vi "_Read File Header.vi"(5 "error in (no error)":errorcluster, 7 "File Size":i64, 8 "File Refnum In":refnum<file>) -> (0 "error out":errorcluster, 1 "Version":i32, 2 "Offsets":i64[](array[numeric]), 3 "File Refnum Out":refnum<file>, 4 "AcqMethod":T1[](array[typedef]) {"ScanType" format="%#.6g"; "Mass Range"."Res" items=["High/High", "Medium/Medium", "Low/Low", "High/Medium", "High/Low", "Medium/High", "Medium/Low", "Low/High", "Low/Medium"]})   [LabVIEW 2015]
uses:
  Type/_XML Expt.ctl
  Type/_XML Lens.ctl
  Type/_Mass Range Property.ctl
  Type/_Mass Range Parameters.ctl
  Type/_RT Res Type.ctl
  Type/_GUI Method.ctl
  Type/_Lens Property.ctl
  Type/_Run Mode.ctl
  Configuration/_Global Configuration.vi
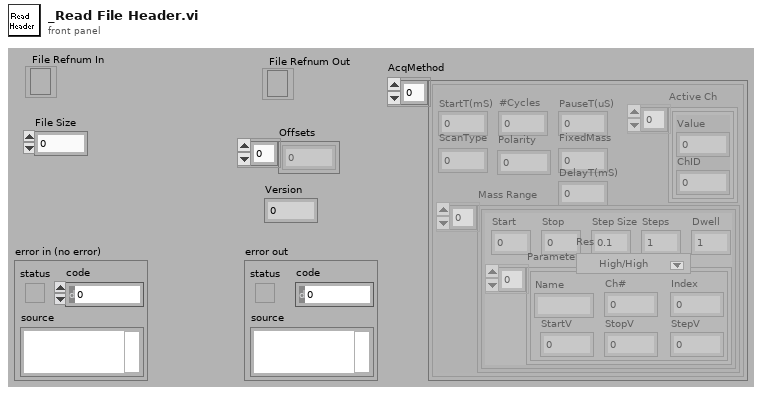
[diagram p1: front panel]
types:
  T1 = typedef "_XML Expt.ctl" = cluster{"StartT(mS)":i32, "#Cycles":i32, "PauseT(uS)":i32, "ScanType":i32, "Polarity":u8, "FixedMass":dbl, "DelayT(mS)":i32, "Active Ch":T2[], "Mass Range":T3[]}
  T2 = typedef "_XML Lens.ctl" = cluster{"Value":dbl, "ChID":u8}
  T3 = typedef "_Mass Range Property.ctl" = cluster{"Start":dbl, "Stop":dbl, "Step Size":dbl, "Steps":i32, "Dwell":dbl, "Parameters":T4[], "Res":T5}
  T4 = typedef "_Mass Range Parameters.ctl" = cluster{"Name":string, "Ch#":u8, "StartV":dbl, "StopV":dbl, "StepV":dbl, "Index":u8}
  T5 = typedef "_RT Res Type.ctl" = u16
  T6 = typedef "_GUI Method.ctl" = cluster{"Lenses":T7[], "Mass Ranges":T3[], "Acquire":bool, "MCA":bool, "Q1DC EN":bool, "Q1 POL":bool, "Q3 POL":bool, "Q1 RF  EN":bool, "Averaging":bool, "Log Scale":bool, "CPS":bool, "Unit":bool, "Data Path":path, "Run Mode":T8, "Fixed Mass (amu)":dbl, "Q3DC EN":bool, "Q3 RF  EN":bool, "Negative":bool}
  T7 = typedef "_Lens Property.ctl" = cluster{"Scan Type":u8, "Scans":i32, "Time 1":dbl, "Time 2":dbl, "Value 1":dbl, "Value 2":dbl, "Step Size":dbl}
  T8 = typedef "_Run Mode.ctl" = enum16{"MRM (Q1/Q2)", "Q1 Scan", "Q1 SRM", "Q2 Scan", "Q2 SRM", "Product Scan", "Precursor Scan", "Neutral Loss", "Neutral Gain"}
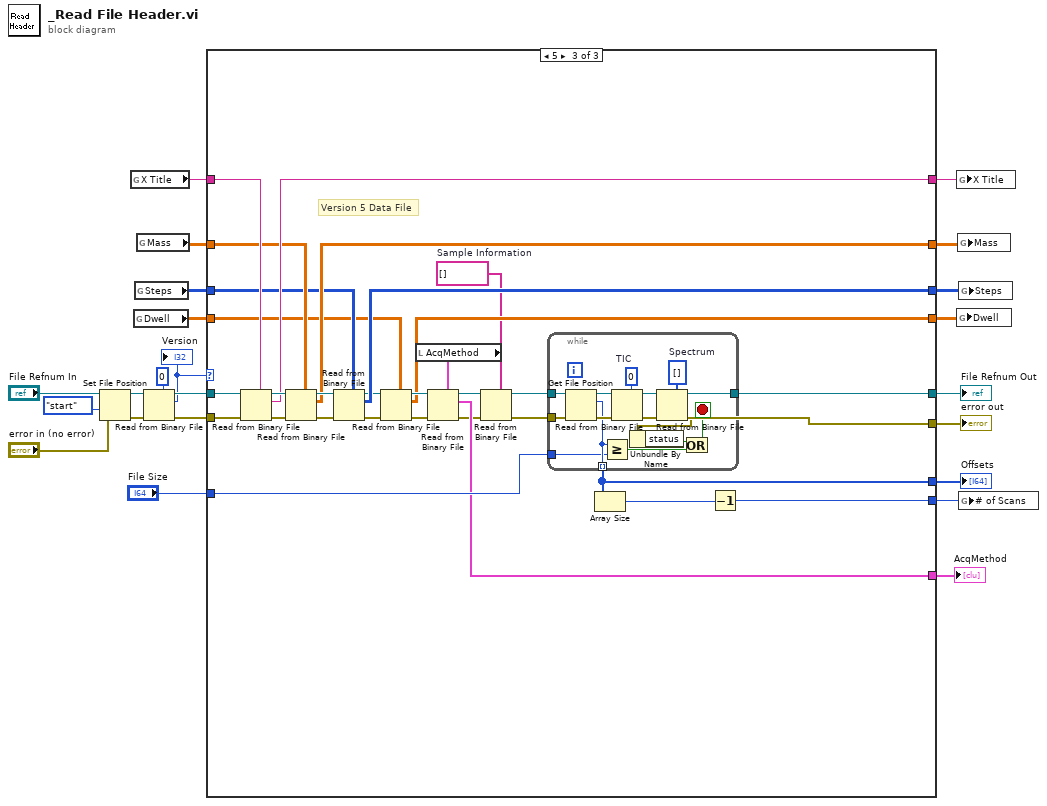
[diagram p0: block diagram]
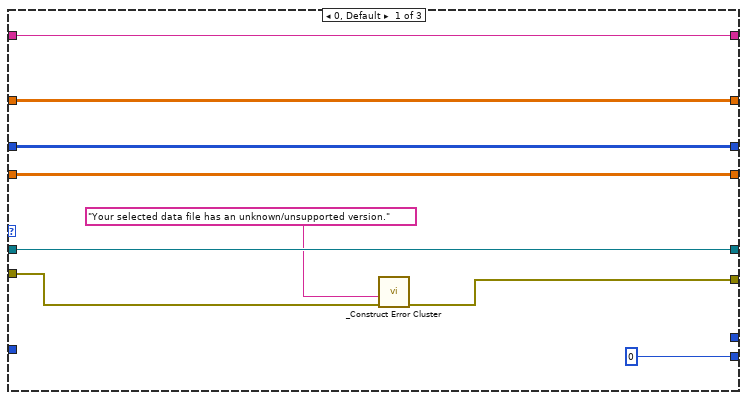
[diagram p2: hidden frame]
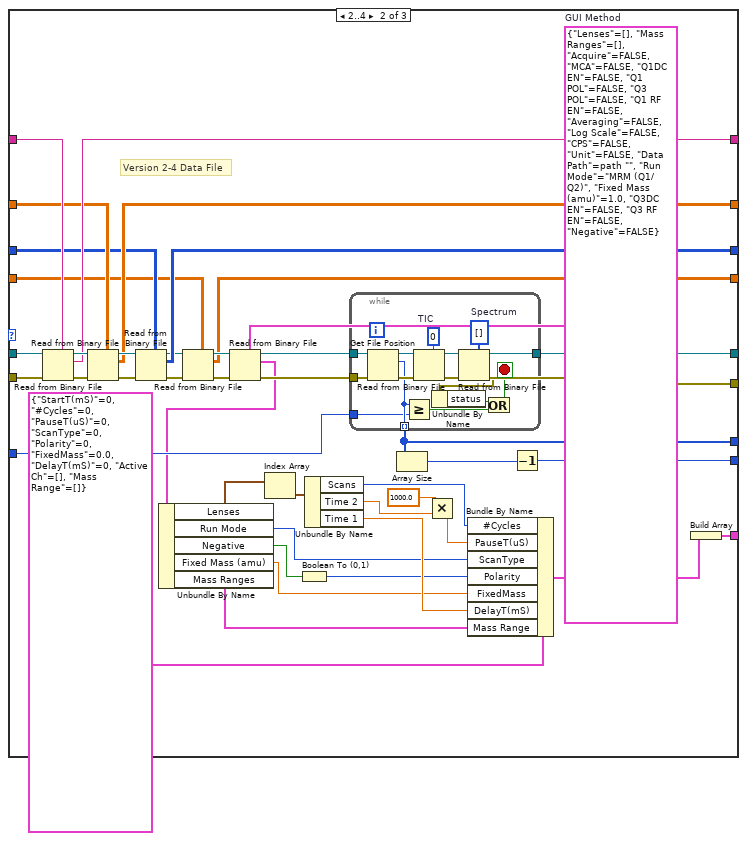
[diagram p3: hidden frame]
diagram:
  n1 = Set File Position(refnum="File Refnum In", from (0:start)=enum16{"start", "end", "current"}."start" ("pos mode (0:2)"), error in="error in (no error)") -> (refnum out=w16:refnum<file>, error out=w15:errorcluster)  [unwired: 1 in]
  n2 = global read "_Global Configuration.vi" "X Title"() -> (w7:string)
  n3 = global read "_Global Configuration.vi" "Dwell"() -> (w4:dbl[][])
  n4 = global read "_Global Configuration.vi" "Steps"() -> (w5:i32[][])
  n5 = global read "_Global Configuration.vi" "Mass"() -> (w6:dbl[][])
  n6 = Read from Binary File(5:0 ("pos offset (0)"), 8:w15, 11:w16) -> (0:w21:errorcluster, 2:w14:i32, 3:w20:refnum<file>)  [unwired: 4 out]
  "Version" <- w14
  n7 = case shown="5" w14 {
    tunnel: w21 -> [w28 w72 w117]
    tunnel: w20 -> [w29 w71 w116]
    tunnel: [w31 w68 w113] -> w17
    tunnel: [w32 w66 w111] -> w13
    tunnel: [0 w51 w98] -> w12
    tunnel: [w29 w55 w101] -> w11
    tunnel: [w26 w54 w92] -> w10
    tunnel: "File Size" -> [_ w50 w97]
    tunnel: [w30 w67 w112] -> w8
    tunnel: w7 -> [w32 w65 w110]
    tunnel: w6 -> [w31 w64 w109]
    tunnel: w5 -> [w30 w63 w108]
    tunnel: w4 -> [w25 w57 w103]
    tunnel: [w25 w56 w102] -> w3
    tunnel: [_ w53 w100] -> w2
    tunnel: [_ w46 w96] -> w1
    frame 0, Default {
      n8 = call "_Construct Error Cluster.vi"("error in"=w28, "reason"="Your selected data file has an unknown/unsupported version.") -> ("error out"=w26:errorcluster)  [unwired: 2 in, 3 out]
    }
    frame 2..4 {
      w49 = T6 {"Lenses"=[], "Mass Ranges"=[], "Acquire"=FALSE, "MCA"=FALSE, "Q1DC EN"=FALSE, "Q1 POL"=FALSE, "Q3 POL"=FALSE, "Q1 RF  EN"=FALSE, "Averaging"=FALSE, "Log Scale"=FALSE, "CPS"=FALSE, "Unit"=FALSE, "Data Path"=path "", "Run Mode"=enum."MRM (Q1/Q2)", "Fixed Mass (amu)"=1.0, "Q3DC EN"=FALSE, "Q3 RF  EN"=FALSE, "Negative"=FALSE}  # GUI Method
      # "Version 2-4 Data File"
      n9 = Read from Binary File(5:w65, 8:w72, 11:w71) -> (0:w74:errorcluster, 2:w66:string, 3:w70:refnum<file>)  [unwired: 4 out]
      n10 = Read from Binary File(5:w64, 8:w74, 11:w70) -> (0:w73:errorcluster, 2:w68:dbl[][], 3:w69:refnum<file>)  [unwired: 4 out]
      n11 = Read from Binary File(5:w63, 8:w73, 11:w69) -> (0:w59:errorcluster, 2:w67:i32[][], 3:w60:refnum<file>)  [unwired: 4 out]
      n12 = Read from Binary File(5:w57, 8:w59, 11:w60) -> (0:w61:errorcluster, 2:w56:dbl[][], 3:w58:refnum<file>)  [unwired: 4 out]
      n13 = Read from Binary File(5:w49, 8:w61, 11:w58) -> (0:w54:errorcluster, 2:w45:T6, 3:w62:refnum<file>)  [unwired: 4 out]
      n14 = Unbundle By Name(w45) -> ("Lenses"=w44:T7[], "Run Mode"=w37:T8, "Negative"=w36:bool, "Fixed Mass (amu)"=w34:dbl, "Mass Ranges"=w33:T3[])
      n15 = Index Array(array=w44) -> (element=w43:T7)  [unwired: 1 in]
      n16 = Boolean To (0,1)(Boolean=w36) -> (0, 1=w35:i16)
      n17 = Unbundle By Name(w43) -> ("Scans"=w42:i32, "Time 2"=w40:dbl, "Time 1"=w38:dbl)
      n18 = while {
        tunnel: w62 -> [w89]
        tunnel: w54 -> [w88]
        tunnel: [w86] -> w55
        tunnel: [w85] -> w53 mode=indexing
        tunnel: w50 -> [w84]
        stop <- w81 stop-if-true
        w76 = u32 0  # TIC
        w87 = u32[] []  # Spectrum
        n19 = Get File Position(4:w88, 7:w89) -> (0:w77:errorcluster, 2:w85:i64, 3:w79:refnum<file>)
        n20 = Greater Or Equal?(x=w85, y=w84) -> (x >= y?=w82:bool)
        n21 = Read from Binary File(5:w76, 8:w77, 11:w79) -> (0:w80:errorcluster, 3:w78:refnum<file>)  [unwired: 5 out]
        n22 = Read from Binary File(5:w87, 8:w80, 11:w78) -> (0:w75:errorcluster, 3:w86:refnum<file>)  [unwired: 5 out]
        n23 = Unbundle By Name(w75) -> ("status"=w83:bool)
        n24 = Or(x=w83, y=w82) -> (x .or. y?=w81:bool)
      }
      n25 = Array Size(array=w53) -> (size(s)=w52:i32)
      n26 = Multiply(x=1000.0 ("y"), y=w40) -> (x*y=w39:dbl)
      n27 = Bundle By Name(cluster=T1 {"StartT(mS)"=0, "#Cycles"=0, "PauseT(uS)"=0, "ScanType"=0, "Polarity"=0, "FixedMass"=0.0, "DelayT(mS)"=0, "Active Ch"=[], "Mass Range"=[]} ("Expt"), "#Cycles"=w42, "PauseT(uS)"=w39, "ScanType"=w37, "Polarity"=w35, "FixedMass"=w34, "DelayT(mS)"=w38, "Mass Range"=w33) -> (w47:T1)
      n28 = Decrement(x=w52) -> (x-1=w51:i32)
      n29 = Build Array(w47) -> (w46:T1[])
    }
    frame 5 {
      w91 = string[] []  # Sample Information
      # "Version 5 Data File"
      n30 = Read from Binary File(5:w110, 8:w117, 11:w116) -> (0:w119:errorcluster, 2:w111:string, 3:w115:refnum<file>)  [unwired: 4 out]
      n31 = Read from Binary File(5:w109, 8:w119, 11:w115) -> (0:w118:errorcluster, 2:w113:dbl[][], 3:w114:refnum<file>)  [unwired: 4 out]
      n32 = Read from Binary File(5:w108, 8:w118, 11:w114) -> (0:w105:errorcluster, 2:w112:i32[][], 3:w106:refnum<file>)  [unwired: 4 out]
      n33 = Read from Binary File(5:w103, 8:w105, 11:w106) -> (0:w107:errorcluster, 2:w102:dbl[][], 3:w104:refnum<file>)  [unwired: 4 out]
      n34 = local read "AcqMethod"() -> (w90:T1[])
      n35 = Read from Binary File(5:w90, 8:w107, 11:w104) -> (0:w95:errorcluster, 2:w96:T1[], 3:w94:refnum<file>)  [unwired: 4 out]
      n36 = Read from Binary File(5:w91, 8:w95, 11:w94) -> (0:w92:errorcluster, 3:w93:refnum<file>)  [unwired: 5 out]
      n37 = while {
        tunnel: w93 -> [w134]
        tunnel: w92 -> [w133]
        tunnel: [w131] -> w101
        tunnel: [w130] -> w100 mode=indexing
        tunnel: w97 -> [w129]
        stop <- w126 stop-if-true
        w121 = u32 0  # TIC
        w132 = u32[] []  # Spectrum
        n38 = Get File Position(4:w133, 7:w134) -> (0:w122:errorcluster, 2:w130:i64, 3:w124:refnum<file>)
        n39 = Greater Or Equal?(x=w130, y=w129) -> (x >= y?=w127:bool)
        n40 = Read from Binary File(5:w121, 8:w122, 11:w124) -> (0:w125:errorcluster, 3:w123:refnum<file>)  [unwired: 5 out]
        n41 = Read from Binary File(5:w132, 8:w125, 11:w123) -> (0:w120:errorcluster, 3:w131:refnum<file>)  [unwired: 5 out]
        n42 = Unbundle By Name(w120) -> ("status"=w128:bool)
        n43 = Or(x=w128, y=w127) -> (x .or. y?=w126:bool)
      }
      n44 = Array Size(array=w100) -> (size(s)=w99:i32)
      n45 = Decrement(x=w99) -> (x-1=w98:i32)
    }
  }
  "File Refnum Out" <- w11
  "error out" <- w10
  "Offsets" <- w2
  "AcqMethod" <- w1
  n46 = global write "_Global Configuration.vi" "X Title"(w13) -> ()
  n47 = global write "_Global Configuration.vi" "Dwell"(w3) -> ()
  n48 = global write "_Global Configuration.vi" "Mass"(w17) -> ()
  n49 = global write "_Global Configuration.vi" "Steps"(w8) -> ()
  n50 = global write "_Global Configuration.vi" "# of Scans"(w12) -> ()
